vi "auto extend.vi"(4 "Hook Motor":T1={"DeviceStatus"={"status"=FALSE, "code"=0, "source"=""}, "Type"=enum."PWM", "PWM"={"PWM Channel"=enum."Invalid", "DeadBand"={"Name"="", "maxPositivePwm"=0, "minPositivePwm"=0, "centerPwm"=0, "maxNegativePwm"=0, "minNegativePwm"=0, "angularRange"=0}}, "CAN"={"Device Number"=0, "Control Mode"=enum."Percent VBus", "Semaphore"=refnum, "Max Vout"=12.0, "TalonSRX Control Mode"=enum."Percent VBus"}, "Invert"=FALSE}, 6 "Scissor Motor":T1={"DeviceStatus"={"status"=FALSE, "code"=0, "source"=""}, "Type"=enum."PWM", "PWM"={"PWM Channel"=enum."Invalid", "DeadBand"={"Name"="", "maxPositivePwm"=0, "minPositivePwm"=0, "centerPwm"=0, "maxNegativePwm"=0, "minNegativePwm"=0, "angularRange"=0}}, "CAN"={"Device Number"=0, "Control Mode"=enum."Percent VBus", "Semaphore"=refnum, "Max Vout"=12.0, "TalonSRX Control Mode"=enum."Percent VBus"}, "Invert"=FALSE}, 9 "Hook Encoder Rate":dbl, 10 "Scissor Encoder Dist":dbl, 11 "Boolean":bool) -> ()   [LabVIEW 2015]
uses:
  <vilib>/Rock Robotics/WPI/MotorControl/WPI_MotorControlDeviceRef.ctl
  <vilib>/Rock Robotics/WPI/MotorControl/WPI_MotorControlType.ctl
  <vilib>/Rock Robotics/SystemInterfaces/DIO/FPGA_DIOPWMChannel.ctl
  <vilib>/Rock Robotics/WPI/PWM/WPI_PWMDeadband.ctl
  <vilib>/Rock Robotics/WPI/CAN/Jaguar/SubVIs/WPI_CANJaguar_ControlMode.ctl
  <vilib>/Rock Robotics/WPI/CAN/TalonSRX/WPI_CANTalonSRX_APIControlMode.ctl
panel:
  in  "Cases":T8(ring)
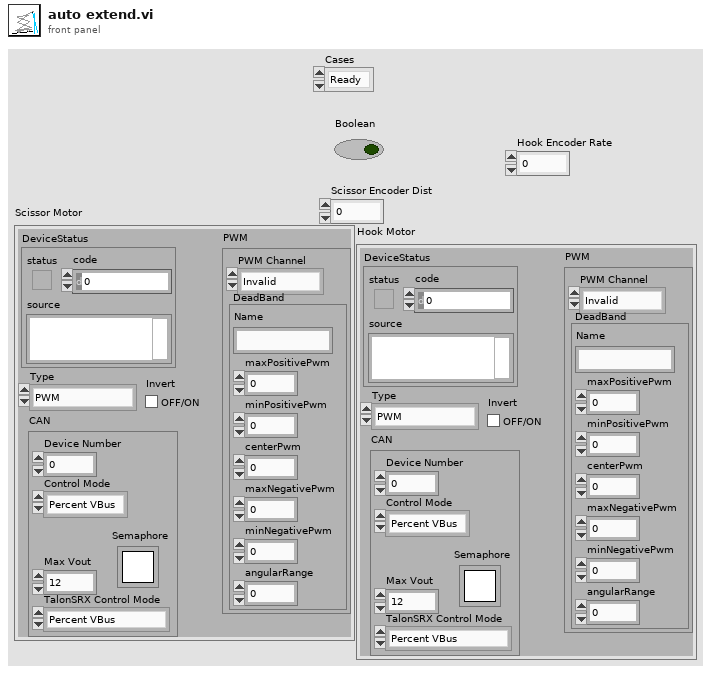
[diagram p1: front panel]
types:
  T1 = typedef "WPI_MotorControlDeviceRef.ctl" = cluster{"DeviceStatus":errorcluster, "Type":T2, "PWM":cluster{"PWM Channel":T3, "DeadBand":T4}, "CAN":cluster{"Device Number":u8, "Control Mode":T5, "Semaphore":T6, "Max Vout":dbl, "TalonSRX Control Mode":T7}, "Invert":bool}
  T2 = typedef "WPI_MotorControlType.ctl" = enum16{"PWM", "CAN", "CANTalonSRX"}
  T3 = typedef "FPGA_DIOPWMChannel.ctl" = enum8{"PWM 0", "PWM 1", "PWM 2", "PWM 3", "PWM 4", "PWM 5", "PWM 6", "PWM 7", "PWM 8", "PWM 9", "PWM MXP 0", "PWM MXP 1", "PWM MXP 2", "PWM MXP 3", "PWM MXP 4", "PWM MXP 5", "PWM MXP 6", "PWM MXP 7", "PWM MXP 8", "PWM MXP 9", "Invalid"}
  T4 = typedef "WPI_PWMDeadband.ctl" = cluster{"Name":string, "maxPositivePwm":i32, "minPositivePwm":i32, "centerPwm":i32, "maxNegativePwm":i32, "minNegativePwm":i32, "angularRange":u16}
  T5 = typedef "WPI_CANJaguar_ControlMode.ctl" = enum8{"Percent VBus", "Current", "Speed", "Position", "Voltage"}
  T6 = typedef "Semaphore RefNum" = refnum<k1>
  T7 = typedef "WPI_CANTalonSRX_APIControlMode.ctl" = enum8{"Percent VBus", "Speed", "Position", "Slave", "Unchanged / Invalid", "Voltage Compensation", "Current", "Motion Profile"}
  T8 = enum16{"Ready", "Extend Lift", "Extend Hook", "Retract Lift", "Hold"}
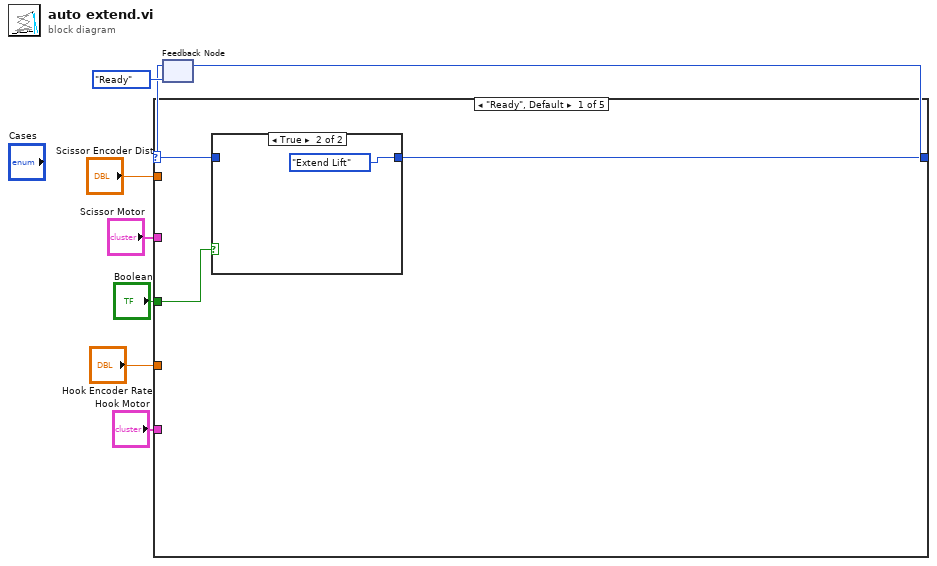
[diagram p0: block diagram]
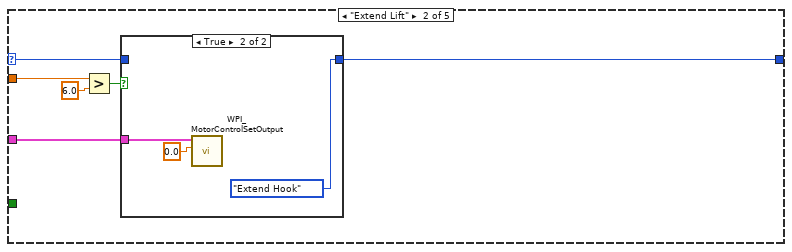
[diagram p3: hidden frame]
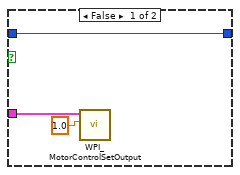
[diagram p4: hidden frame]
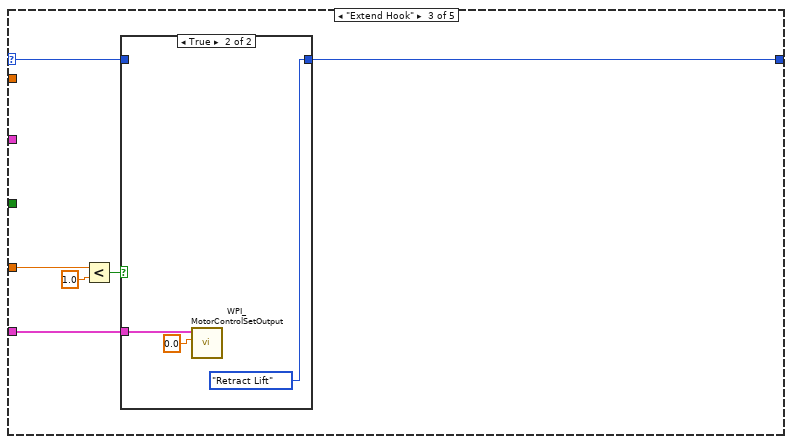
[diagram p5: hidden frame]
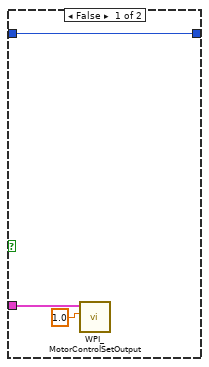
[diagram p6: hidden frame]
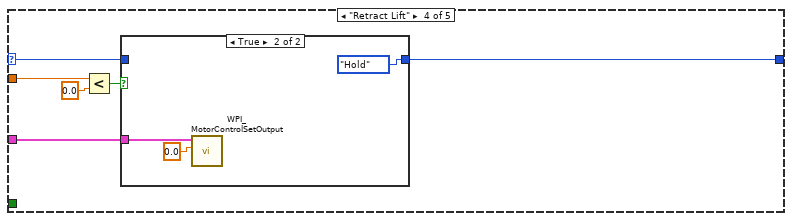
[diagram p7: hidden frame]
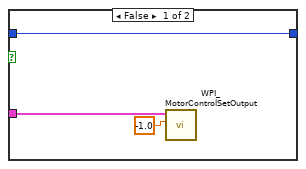
[diagram p8: hidden frame]
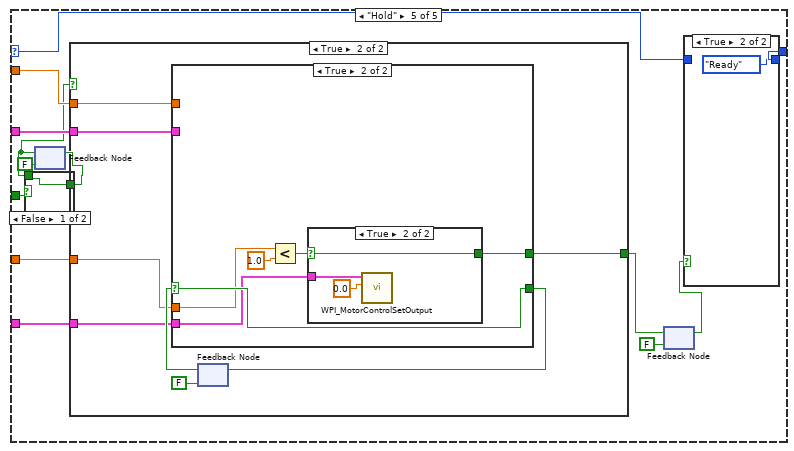
[diagram p9: hidden frame]
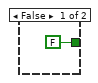
[diagram p11: hidden frame]
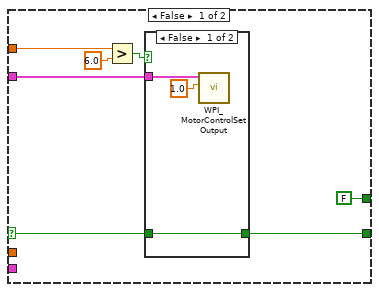
[diagram p12: hidden frame]
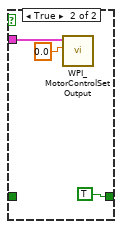
[diagram p13: hidden frame]
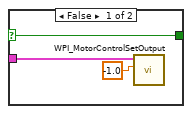
[diagram p14: hidden frame]
diagram:
  n1 = feedback #1(T8."Ready" ("Cases")) -> (w7:T8)
  n2 = case shown="\"Ready\", Default" w7 {
    selector: w7 -> [w11 w18 w31 w43 w62]
    tunnel: [w10 w19 w30 w42 w61] -> w6
    tunnel: "Boolean" -> [w9 _ _ _ w53]
    tunnel: "Scissor Encoder Dist" -> [_ w17 _ w40 w59]
    tunnel: "Scissor Motor" -> [_ w14 _ w41 w58]
    tunnel: "Hook Encoder Rate" -> [_ _ w28 _ w60]
    tunnel: "Hook Motor" -> [_ _ w26 _ w57]
    frame "Ready", Default {
      n3 = case shown="True" w9 {
        tunnel: [w12 T8."Extend Lift" ("Cases")] -> w10
        tunnel: w11 -> [w12 _]
        frame False {
        }
        frame True {
        }
      }
    }
    frame "Extend Lift" {
      n4 = Greater?(x=w17, y=6.0) -> (0:w15:bool)
      n5 = case shown="True" w15 {
        tunnel: [w22 T8."Extend Hook" ("Cases")] -> w19
        tunnel: w18 -> [w22 _]
        tunnel: w14 -> [w20 w23]
        frame False {
          n6 = call <vilib>:"WPI_MotorControlSetOutput.vi"("Output"=1.0, "MotorControlDevRef"=w20) -> ()  [unwired: 7 in, 3 out]
        }
        frame True {
          n7 = call <vilib>:"WPI_MotorControlSetOutput.vi"("Output"=0.0, "MotorControlDevRef"=w23) -> ()  [unwired: 7 in, 3 out]
        }
      }
    }
    frame "Extend Hook" {
      n8 = Less?(x=w28, y=1.0) -> (x < y?=w27:bool)
      n9 = case shown="True" w27 {
        tunnel: [w34 T8."Retract Lift" ("Cases")] -> w30
        tunnel: w31 -> [w34 _]
        tunnel: w26 -> [w33 w36]
        frame False {
          n10 = call <vilib>:"WPI_MotorControlSetOutput.vi"("Output"=1.0, "MotorControlDevRef"=w33) -> ()  [unwired: 7 in, 3 out]
        }
        frame True {
          n11 = call <vilib>:"WPI_MotorControlSetOutput.vi"("Output"=0.0, "MotorControlDevRef"=w36) -> ()  [unwired: 7 in, 3 out]
        }
      }
    }
    frame "Retract Lift" {
      n12 = Less?(x=w40, y=0.0) -> (x < y?=w38:bool)
      n13 = case shown="True" w38 {
        tunnel: [w46 T8."Hold" ("Cases")] -> w42
        tunnel: w43 -> [w46 _]
        tunnel: w41 -> [w44 w47]
        frame False {
          n14 = call <vilib>:"WPI_MotorControlSetOutput.vi"("Output"=-1.0, "MotorControlDevRef"=w44) -> ()  [unwired: 7 in, 3 out]
        }
        frame True {
          n15 = call <vilib>:"WPI_MotorControlSetOutput.vi"("Output"=0.0, "MotorControlDevRef"=w47) -> ()  [unwired: 7 in, 3 out]
        }
      }
    }
    frame "Hold" {
      n16 = feedback #2(FALSE) -> (w50:bool)
      n17 = case shown="False" w53 {
        selector: w53 -> [_ w64]
        tunnel: [w63 w64] -> w52
        tunnel: w50 -> [w63 _]
        frame False {
        }
        frame True {
        }
      }
      n18 = feedback-in #2(w52) -> ()
      n19 = case shown="True" w50 {
        tunnel: w60 -> [_ w68]
        tunnel: w59 -> [_ w70]
        tunnel: w58 -> [_ w69]
        tunnel: w57 -> [_ w67]
        tunnel: [FALSE w66] -> w56
        frame False {
        }
        frame True {
          n20 = feedback #3(FALSE) -> (w73:bool)
          n21 = case shown="True" w73 {
            selector: w73 -> [w79 w92]
            tunnel: [w80 w92] -> w71
            tunnel: w70 -> [w78 _]
            tunnel: w69 -> [w75 _]
            tunnel: w68 -> [_ w91]
            tunnel: w67 -> [_ w89]
            tunnel: [FALSE w87] -> w66
            frame False {
              n22 = Greater?(x=w78, y=6.0) -> (0:w76:bool)
              n23 = case shown="False" w76 {
                tunnel: [w83 TRUE] -> w80
                tunnel: w79 -> [w83 _]
                tunnel: w75 -> [w82 w84]
                frame False {
                  n24 = call <vilib>:"WPI_MotorControlSetOutput.vi"("Output"=1.0, "MotorControlDevRef"=w82) -> ()  [unwired: 7 in, 3 out]
                }
                frame True {
                  n25 = call <vilib>:"WPI_MotorControlSetOutput.vi"("Output"=0.0, "MotorControlDevRef"=w84) -> ()  [unwired: 7 in, 3 out]
                }
              }
            }
            frame True {
              n26 = Less?(x=w91, y=1.0) -> (x < y?=w88:bool)
              n27 = case shown="True" w88 {
                selector: w88 -> [w93 w96]
                tunnel: w89 -> [w95 w98]
                tunnel: [w93 w96] -> w87
                frame False {
                  n28 = call <vilib>:"WPI_MotorControlSetOutput.vi"("Output"=-1.0, "MotorControlDevRef"=w95) -> ()  [unwired: 7 in, 3 out]
                }
                frame True {
                  n29 = call <vilib>:"WPI_MotorControlSetOutput.vi"("Output"=0.0, "MotorControlDevRef"=w98) -> ()  [unwired: 7 in, 3 out]
                }
              }
            }
          }
          n30 = feedback-in #3(w71) -> ()
        }
      }
      n31 = feedback-in #4(w56) -> ()
      n32 = feedback #4(FALSE) -> (w55:bool)
      n33 = case shown="True" w55 {
        tunnel: [w99 T8."Ready" ("Cases")] -> w61
        tunnel: w62 -> [w99 _]
        frame False {
        }
        frame True {
        }
      }
    }
  }
  n34 = feedback-in #1(w6) -> ()
